vi "KE2425_Reverse.vi"(8 "error in (no error)":errorcluster, 11 "Instruments in":refnum<class "Instruments.lvclass">) -> (0 "error out":errorcluster, 2 "Current(A)":dbl format="%0.2f", 3 "Instruments out":refnum<class "Instruments.lvclass">, 7 "Keithley Error":bool)   [LabVIEW 2012, in "Instruments.lvclass"]
uses:
  Instruments.lvclass
  Instruments.lvclass/Instruments.ctl
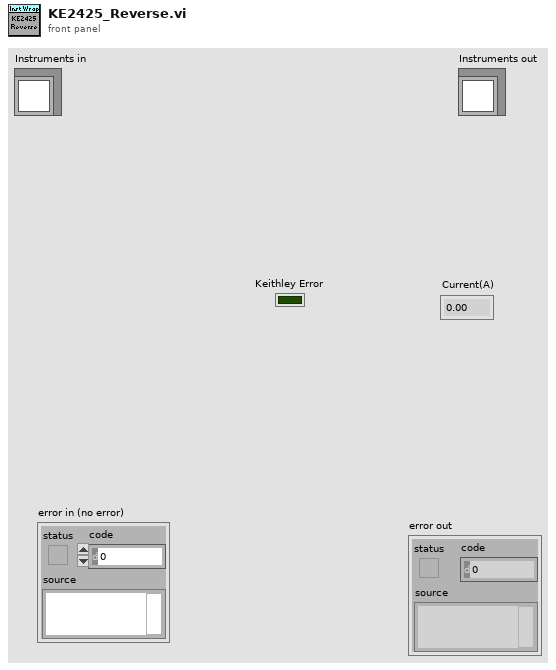
[diagram p1: front panel]
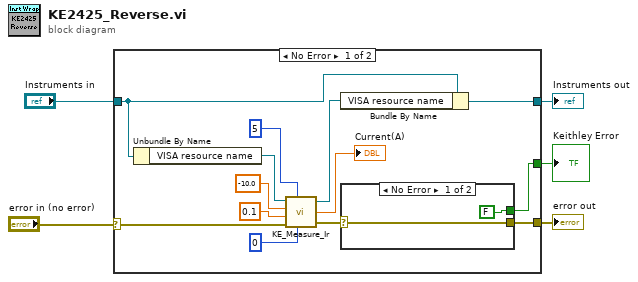
[diagram p0: block diagram]
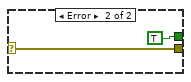
[diagram p2: hidden frame]
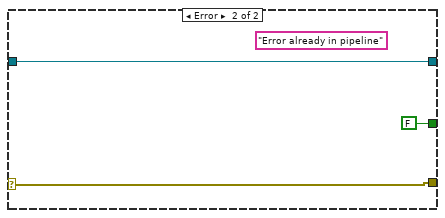
[diagram p3: hidden frame]
diagram:
  n1 = case shown="No Error" "error in (no error)" {
    selector: "error in (no error)" -> [w17 w25]
    tunnel: [w6 w25] -> w4
    tunnel: [w11 w24] -> w2
    tunnel: "Instruments in" -> [w13 w24]
    tunnel: [w7 FALSE] -> w1
    frame No Error {
      n2 = Unbundle By Name(w13) -> ("VISA resource name"=w18:refnum<visa-resource-name>)
      n3 = call "KE_Measure_Ir.vi"("KE_In"=w18, "Samples"=5, "Voltage"=-10.0, "Compliance"=0.1, "SettleDelay"=u32 0, "error in (no error)"=w17) -> ("KE_Out"=w12:refnum<visa-resource-name>, "Current(A)"=→"Current(A)":dbl, "error out"=w8:errorcluster)
      n4 = Bundle By Name(cluster=w13, "VISA resource name"=w12) -> (w11:refnum<class "Instruments.lvclass">)
      n5 = case shown="No Error" w8 {
        selector: w8 -> [w19 w21]
        tunnel: [FALSE TRUE] -> w7
        tunnel: [w19 w21] -> w6
        frame No Error {
        }
        frame Error {
        }
      }
    }
    frame Error {
      (unwired) "Error already in pipeline" ("device dependent errors")
    }
  }
  "error out" <- w4
  "Instruments out" <- w2
  "Keithley Error" <- w1
